vi "MeasAction.vi"(8 "error in (no error)":errorcluster caption="entrée d'erreur (pas d'erreur)", 9 "CurvePointIndex":i32, 10 "AllPointIndex":i32, 11 "InstrClassIn":refnum<class "Agilent34410A.lvclass"> caption="DNL_LabVIEW Object in") -> (0 "error out":errorcluster caption="sortie d'erreur", 2 "MeasDatOut":dbl[](array[numeric]), 3 "InstrClassOut":refnum<class "Agilent34410A.lvclass"> caption="DNL_LabVIEW Object out")   [LabVIEW 2019, in "Agilent34410A.lvclass"]
uses:
  Agilent34410A.lvclass
  C:/Programmes Labview/LabScanV1A/DevicesClass/BaseDevice/BaseDevice.lvclass
  Agilent34410A.lvclass/Agilent34410A.ctl
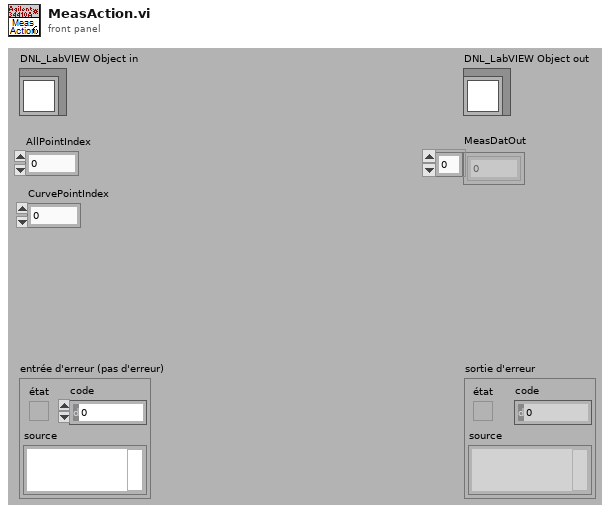
[diagram p1: front panel]
types:
  T1 = typedef "Agilent34410A.lvclass/Agilent34410A_Func.ctl" = enum16{"Read Function (Arb)", "Read Voltage (V)", "Read Current (A)", "Read 2W Resistance (Ohms)", "Read 4W Resistance (Ohms)"}
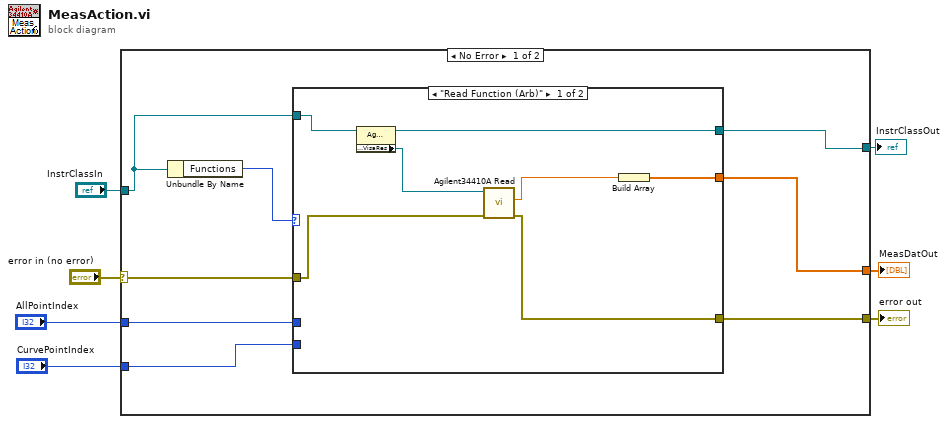
[diagram p0: block diagram]
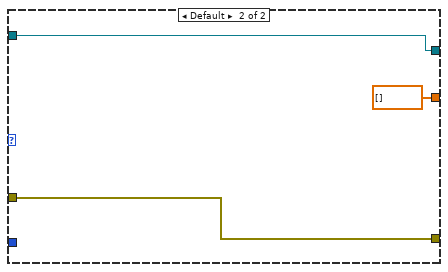
[diagram p2: hidden frame]
diagram:
  n1 = case shown="No Error" "error in (no error)" {
    selector: "error in (no error)" -> [w11 w26]
    tunnel: "InstrClassIn" -> [w9 w27]
    tunnel: [w8 w27] -> w5
    tunnel: "AllPointIndex" -> [w15 _]
    tunnel: [w14 w26] -> w3
    tunnel: [w13 _] -> w2
    tunnel: "CurvePointIndex" -> [w10 _]
    frame No Error {
      n2 = Unbundle By Name(w9) -> ("Functions"=w12:T1)
      n3 = case shown="\"Read Function (Arb)\"" w12 {
        tunnel: w15 -> [_ _]
        tunnel: [w18 w24] -> w14
        tunnel: [w16 dbl[] [] ("Outputs")] -> w13
        tunnel: w11 -> [w19 w24]
        tunnel: w10 -> [_ _]
        tunnel: w9 -> [w22 w23]
        tunnel: [w21 w23] -> w8
        frame "Read Function (Arb)" {
          n4 = property class="Agilent34410A.lvclass"(reference=w22) -> (reference out=w21:refnum<class "Agilent34410A.lvclass">, "Accessor:VisaRes"=w20:refnum<visa-resource-name>)  [unwired: 1 in, 1 out]
          n5 = call <userlib>:"Agilent34410A Read.vi"("error in (no error)"=w19, "VISA Rsrc"=w20) -> ("error out"=w18:errorcluster, "Reading"=w17:dbl)  [unwired: 6 in, 2 out]
          n6 = Build Array(w17) -> (w16:dbl[])
        }
        frame Default {
        }
      }
    }
    frame Error {
    }
  }
  "error out" <- w3
  "InstrClassOut" <- w5
  "MeasDatOut" <- w2
